vi "RWpbData.vi"(4 "error in (no error)":errorcluster, 6 "TXSTR":string, 7 "VISA resource":refnum<visa-resource-name>="COM1") -> (0 "error out":errorcluster, 2 "RXSTR":string, 3 "dup VISA resource":refnum<visa-resource-name>="COM1")   [LabVIEW 2021]
doc: "Reads and writes data\nto/from AVS-47B"
panel:
  out "OUTSTR":string="0000000000"
  # "RWpbData.vi"
  # "Sends the Picobus Address (PBA) to the AVS-47B. All Picobus transactions with the bridge \nconsist of the following sequence:\n\n1) send Picobus address (8 bits)\n2) strobe the address\n3) send and read data (48 bits)\n4) strobe the data\n\nEvery transaction contains both writing (a possibly new) configuration and reading the \nexisting (old) configuration from the bridge. Together with the configuration, the AVS-47B \nsends also the result of the latest A/D conversion to the PC.  Reading the conversion result \ndoes not reset it."
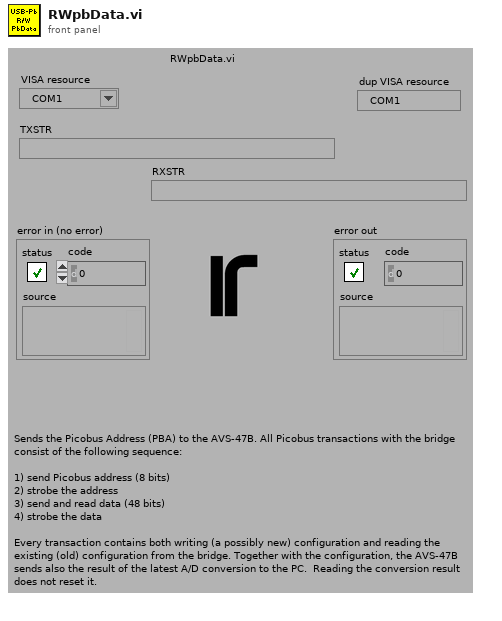
[diagram p1: front panel]
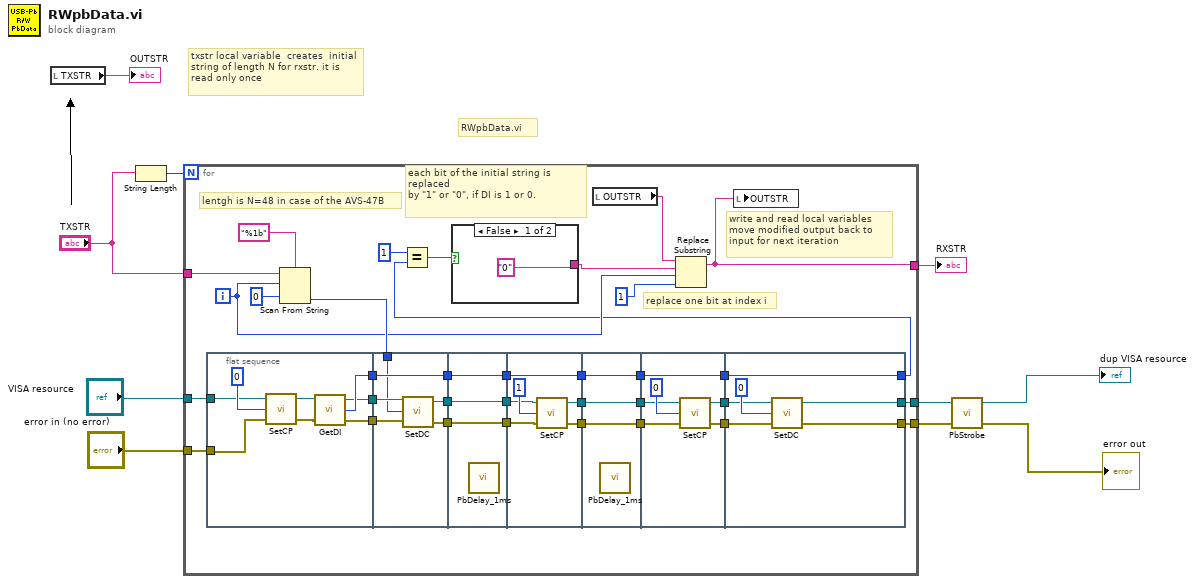
[diagram p0: block diagram]
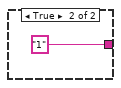
[diagram p2: hidden frame]
diagram:
  # "RWpbData.vi"
  # "txstr local variable  creates  initial string of length N for rxstr. it is read only once"
  n1 = local read "TXSTR"() -> (→"OUTSTR":string)
  n2 = String Length(string="TXSTR") -> (length=w10:i32)
  n3 = for {
    N: w10 -> [_]
    tunnel: "TXSTR" -> [w38]
    tunnel: [w34] -> w8
    tunnel: "VISA resource" -> [w26]
    tunnel: "error in (no error)" -> [w19]
    tunnel: [w12] -> w5
    tunnel: [w11] -> w4
    i -> [w37]
    # "lentgh is N=48 in case of the AVS-47B"
    # "replace one bit at index i"
    # "each bit of the initial string is replaced\nby \"1\" or \"0\", if DI is 1 or 0."
    # "write and read local variables\nmove modified output back to\ninput for next iteration"
    n4 = flat-sequence {
      tunnel: [w54] -> w27
      tunnel: w26 -> [w52]
      tunnel: [w50] -> w25
      tunnel: w19 -> [w47]
      tunnel: [w48] -> w18
      tunnel: w44 -> [w55]
      tunnel: [w60] -> w28
      tunnel: w27 -> [w60]
      tunnel: w25 -> [w59]
      tunnel: [w58] -> w23
      tunnel: w18 -> [w57]
      tunnel: [w56] -> w16
      tunnel: [w63] -> w29
      tunnel: w28 -> [w63]
      tunnel: [w62] -> w24
      tunnel: w23 -> [w62]
      tunnel: [w61] -> w17
      tunnel: w16 -> [w61]
      tunnel: [w69] -> w30
      tunnel: w29 -> [w69]
      tunnel: w24 -> [w67]
      tunnel: [w66] -> w21
      tunnel: w17 -> [w65]
      tunnel: [w64] -> w14
      tunnel: [w72] -> w31
      tunnel: w30 -> [w72]
      tunnel: [w71] -> w22
      tunnel: w21 -> [w71]
      tunnel: [w70] -> w15
      tunnel: w14 -> [w70]
      tunnel: [w78] -> w32
      tunnel: w31 -> [w78]
      tunnel: w22 -> [w76]
      tunnel: [w75] -> w20
      tunnel: w15 -> [w74]
      tunnel: [w73] -> w13
      tunnel: [w84] -> w33
      tunnel: w32 -> [w84]
      tunnel: w20 -> [w82]
      tunnel: w13 -> [w81]
      tunnel: [w80] -> w12
      tunnel: [w79] -> w11
      frame #0 {
        n5 = call "SetCP.vi"("error in (no error)"=w47, "CP(=RTS) state"=u8 0, "VISA resource"=w52) -> ("error out"=w49:errorcluster, "dup VISA resource"=w51:refnum<visa-resource-name>)  [unwired: 1 in]
        n6 = call "GetDI.vi"("error in (no error)"=w49, "VISA resource"=w51) -> ("error out"=w48:errorcluster, "DI(=CTS) State"=w54:i16, "dup VISA resource"=w50:refnum<visa-resource-name>)  [unwired: 1 in]
      }
      frame #1 {
        n7 = call "SetDC.vi"("error in (no error)"=w57, "DC(=DTR) state"=w55, "VISA resource"=w59) -> ("error out"=w56:errorcluster, "dup VISA resource"=w58:refnum<visa-resource-name>)  [unwired: 1 in]
      }
      frame #2 {
        n8 = call "PbDelay_1ms.vi"() -> ()  [unwired: 4 in]
      }
      frame #3 {
        n9 = call "SetCP.vi"("error in (no error)"=w65, "CP(=RTS) state"=u8 1, "VISA resource"=w67) -> ("error out"=w64:errorcluster, "dup VISA resource"=w66:refnum<visa-resource-name>)  [unwired: 1 in]
      }
      frame #4 {
        n10 = call "PbDelay_1ms.vi"() -> ()  [unwired: 4 in]
      }
      frame #5 {
        n11 = call "SetCP.vi"("error in (no error)"=w74, "CP(=RTS) state"=u8 0, "VISA resource"=w76) -> ("error out"=w73:errorcluster, "dup VISA resource"=w75:refnum<visa-resource-name>)  [unwired: 1 in]
      }
      frame #6 {
        n12 = call "SetDC.vi"("error in (no error)"=w81, "DC(=DTR) state"=u8 0, "VISA resource"=w82) -> ("error out"=w79:errorcluster, "dup VISA resource"=w80:refnum<visa-resource-name>)  [unwired: 1 in]
      }
    }
    n13 = Scan From String(format string="%1b", input string=w38, initial scan location=w37, default 1=u8 0) -> (output 1=w44:u8)  [unwired: 1 in, 3 out]
    n14 = Equal?(x=u8 1, y=w33) -> (x = y?=w40:bool)
    n15 = case shown="False" w40 {
      tunnel: ["0" "1"] -> w39
      frame False {
      }
      frame True {
      }
    }
    n16 = local read "OUTSTR"() -> (w35:string)
    n17 = Replace Substring(2:u8 1, 3:w37, 4:w39, 5:w35) -> (1:w34:string)  [unwired: 1 out]
    n18 = local write "OUTSTR"(w34) -> ()
  }
  "RXSTR" <- w8
  n19 = call "PbStrobe.vi"("error in (no error)"=w4, "VISA resource"=w5) -> ("error out"=→"error out":errorcluster, "dup VISA resource"=→"dup VISA resource":refnum<visa-resource-name>)  [unwired: 2 in]
